vi "Launch Progress Bar.vi"(7 "Calling VI Ref":refnum<vi>, 8 "error in (no error)":errorcluster, 9 "Enable Cancellation? (T)":bool=TRUE, 10 "Main Title (\"Loading item data...\")":string="Loading item data...", 11 "Total Count":i32) -> (0 "error out":errorcluster, 3 "Progress Bar Dialog":refnum<class "Loading Dialog.lvclass">)   [LabVIEW 2020, in "VI Properties Editor.lvlib" / "Loading Dialog.lvclass"]
doc: "Creates an instance of a progress bar dialog and sets the total number of steps that are expected to be performed. Note that the window will not appear until 500ms have passed in order to avoid rapidly flashing the window during repeated quick sequences."
uses:
  Loading Dialog.lvclass
  Loading Dialog.lvclass/Loading Dialog.ctl
  Progress Bar Front Panel.vi
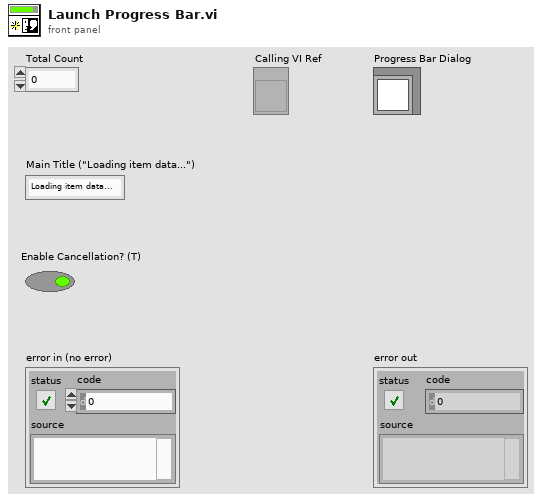
[diagram p1: front panel]
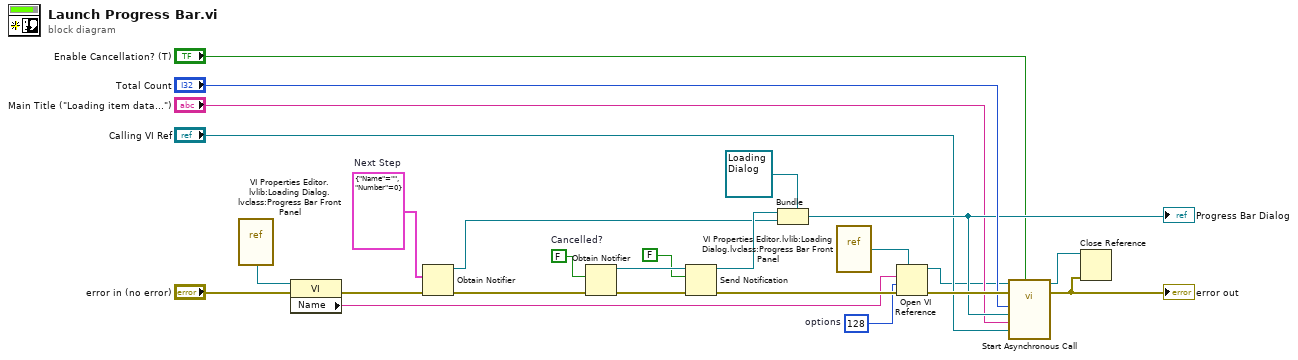
[diagram p0: block diagram]
diagram:
  w2 = cluster{"Name":string, "Number":i32} {"Name"="", "Number"=0}  # Next Step
  w7 = FALSE  # Cancelled?
  w10 = 128  # options
  n1 = vi-ref "VI Properties Editor.lvlib:Loading Dialog.lvclass:Progress Bar Front Panel.vi"() -> (w11:refnum<vi>)
  n2 = property class="VI"(reference=w11, error in="error in (no error)") -> (error out=w22:errorcluster, "Name"=w12:string)  [unwired: 1 out]
  n3 = Obtain Notifier(notification data type=w2, error in (no error)=w22) -> (notifier out=w1:refnum<notifier>, error out=w21:errorcluster)  [unwired: 2 in, 1 out]
  n4 = Obtain Notifier(notification data type=w7, error in (no error)=w21) -> (notifier out=w18:refnum<notifier>, error out=w20:errorcluster)  [unwired: 2 in, 1 out]
  n5 = Send Notification(notification=FALSE, notifier=w18, error in (no error)=w20) -> (notifier out=w5:refnum<notifier>, error out=w19:errorcluster)
  n6 = Bundle(cluster=refnum<class "Loading Dialog.lvclass"> refnum ("Progress Bar Dialog"), w5, w1) -> (w16:refnum<class "Loading Dialog.lvclass">)
  "Progress Bar Dialog" <- w16
  n7 = vi-ref "VI Properties Editor.lvlib:Loading Dialog.lvclass:Progress Bar Front Panel.vi"() -> (w8:refnum<vi>)
  n8 = Open VI Reference(type specifier VI Refnum (for type only)=w8, vi path=w12, options=w10, error in (no error)=w19) -> (vi reference=w9:refnum<vi>, error out=w23:errorcluster)  [unwired: 2 in]
  n9 = call-by-ref "Start Asynchronous Call"(reference=w9, error in=w23, "Enable Cancel?"="Enable Cancellation? (T)", "Calling VI Ref"="Calling VI Ref", "Main Title"="Main Title (\"Loading item data...\")", "Progress Bar Dialog"=w16, "Total"="Total Count") -> (reference out=w3:refnum<vi>, error out=w25:errorcluster)  [unwired: 7 in]
  "error out" <- w25
  n10 = Close Reference(reference=w3, error in (no error)=w25) -> ()  [unwired: 1 out]
